vi "_CSMOFGV Dequeue.vi"(8 "Error In":errorcluster caption="error in (no error)", 9 "Dequeue Timeout (0ms)":i32, 10 "State (S) In (\"\")":string, 11 "CSMQ In":T1={"info"={"Module Name"="", "Requested Name"="", "Group Name"="", "Mode"=enum."Stand Alone", "Allowed Messages"=[]}, "Refs"={"WatchDogQ"=refnum, "CSMDataDVR"=refnum, "Queue"={"HPriorityQ"=refnum, "LowPriorityQ"=refnum}, "GroupDataDVR"=refnum, "TagMap"=refnum, "ExitEvent"=refnum, "NewStateEvent"=refnum, "StatusChangeEvent"=refnum}}) -> (0 "error out":errorcluster, 2 "States Out":string, 3 "CSMQ Out":T1={"info"={"Module Name"="", "Requested Name"="", "Group Name"="", "Mode"=enum."Stand Alone", "Allowed Messages"=[]}, "Refs"={"WatchDogQ"=refnum, "CSMDataDVR"=refnum, "Queue"={"HPriorityQ"=refnum, "LowPriorityQ"=refnum}, "GroupDataDVR"=refnum, "TagMap"=refnum, "ExitEvent"=refnum, "NewStateEvent"=refnum, "StatusChangeEvent"=refnum}})   [LabVIEW 2017, in "Communicable State Machine.lvlib"]
uses:
  Communicable State Machine.lvlib
  _CSMObj.ctl
  _CSMObj-Info.ctl
  Typedef/_CSM_MODE.ctl
  _CSMObj-Refs.ctl
  _CSMObj-Data.ctl
  Priority Queue/Priority Queue.ctl
  Typedef/_Cross CSM State Data.ctl
  Typedef/_CSM_MSG_TYPE.ctl
  Typedef/_Cross CSM State Response.ctl
  Typedef/_CSM_Response Source Message.ctl
  Priority Queue/def-Data(LowPRI-Q).ctl
  _CSMObj-ModeData.ctl
  Typedef/_CSM Status Change Event Data.ctl
  AdvanceAPI/CSM - Make String Arguments Safe.vi
  AdvanceAPI/CSM - Keywords.vi
  _Shared/CSM Shared.lvlib
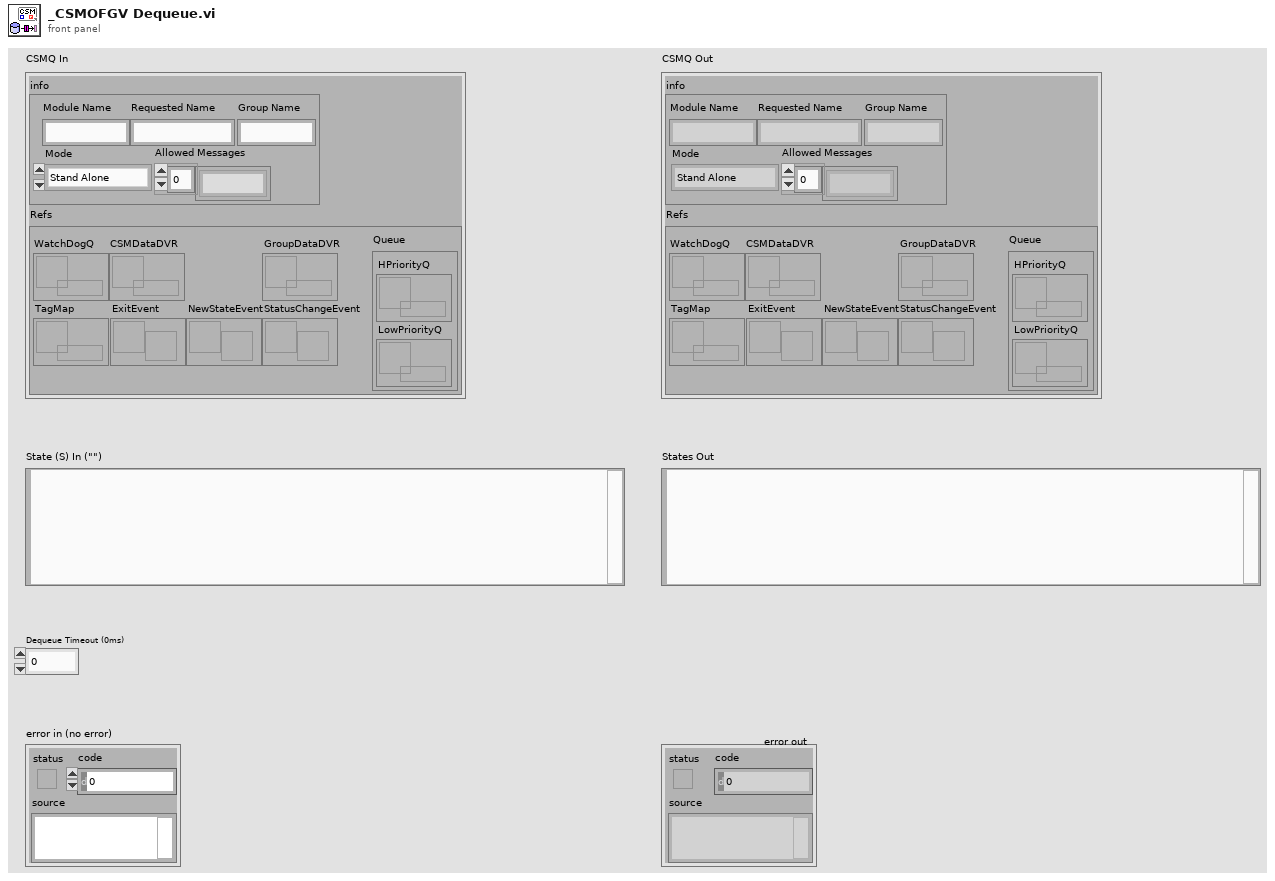
[diagram p1: front panel]
types:
  T1 = typedef "Communicable State Machine.lvlib/_CSMObj.ctl" = cluster{"info":T2, "Refs":T4}
  T2 = typedef "Communicable State Machine.lvlib/_CSMObj-Info.ctl" = cluster{"Module Name":string, "Requested Name":string, "Group Name":string, "Mode":T3, "Allowed Messages":string[]}
  T3 = typedef "Communicable State Machine.lvlib/_CSM_MODE.ctl" = enum16{"Not Exist", "Stand Alone", "CSM", "Worker", "Worker Agent", "Chain Node", "Chain"}
  T4 = typedef "Communicable State Machine.lvlib/_CSMObj-Refs.ctl" = cluster{"WatchDogQ":refnum<queue>, "CSMDataDVR":refnum<data-value>, "Queue":T5, "GroupDataDVR":refnum<data-value>, "TagMap":refnum<data-value>, "ExitEvent":refnum<user-event>, "NewStateEvent":refnum<user-event>, "StatusChangeEvent":refnum<user-event>}
  T5 = typedef "Communicable State Machine.lvlib/Priority Queue.ctl" = cluster{"HPriorityQ":refnum<queue>, "LowPriorityQ":refnum<queue>}
  T6 = typedef "Communicable State Machine.lvlib/_CSMObj-Data.ctl" = cluster{"RemoteMessge?":bool, "error":errorcluster, "InternalRegistryRules":string[], "Return State":string, "Initialized":enum16{"Initializing", "Ready", "Exiting"}}
  T7 = typedef "Communicable State Machine.lvlib/_Cross CSM State Data.ctl" = cluster{"Msg Type":T8, "state":string, "args":string, "source":string, "RespQ":refnum<queue>, "Response For Message":T9, "Target":string}
  T8 = typedef "Communicable State Machine.lvlib/_CSM_MSG_TYPE.ctl" = enum16{"Sync Message(-@)", "Async Message(->)", "Async without Response(->|)", "Async Response", "Broadcast(-><all>)", "Broadcast(-><status>)", "Broadcast(-><interrupt>)", "Append to JKISM States", "Append to JKISM States(High Priority)", "Broadcast(-><state>)"}
  T9 = typedef "Communicable State Machine.lvlib/_CSM_Response Source Message.ctl" = cluster{"‘State":string, "’Arguments":string, "’Error":errorcluster}
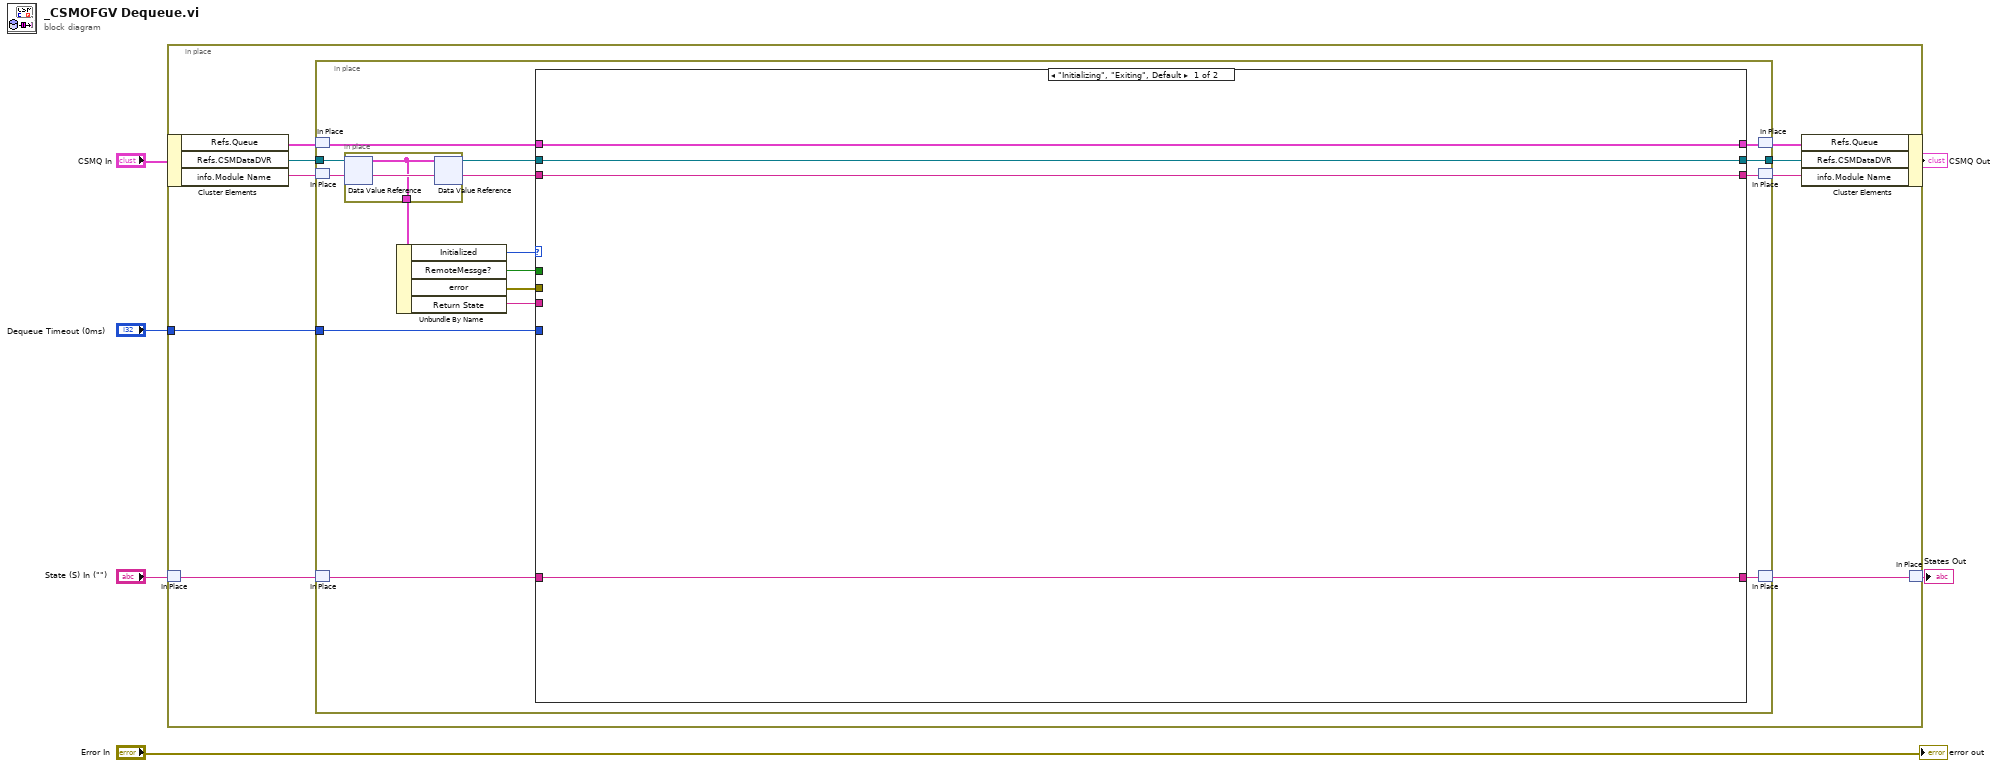
[diagram p0: block diagram]
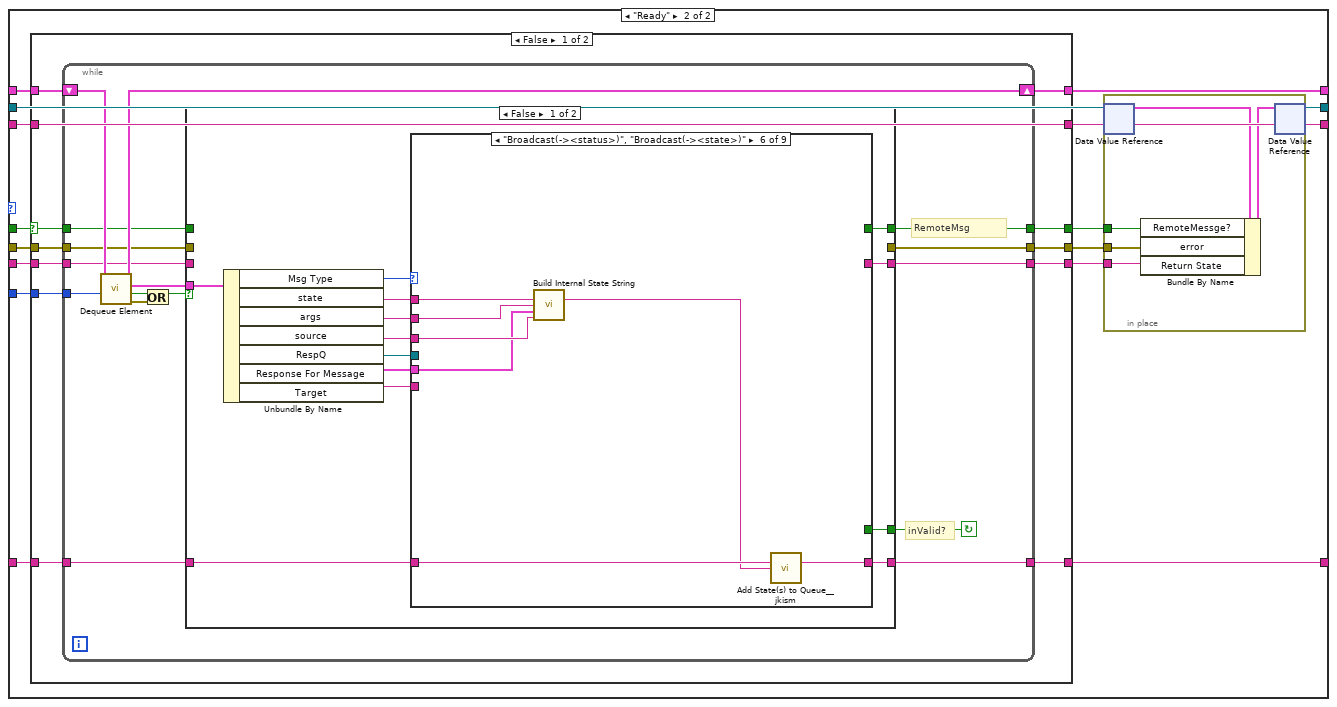
[diagram p2: hidden frame]
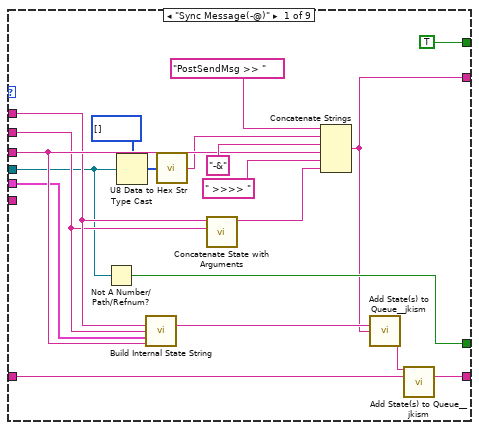
[diagram p3: hidden frame]
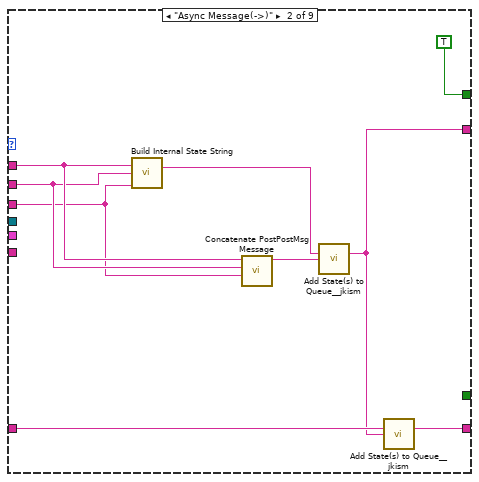
[diagram p4: hidden frame]
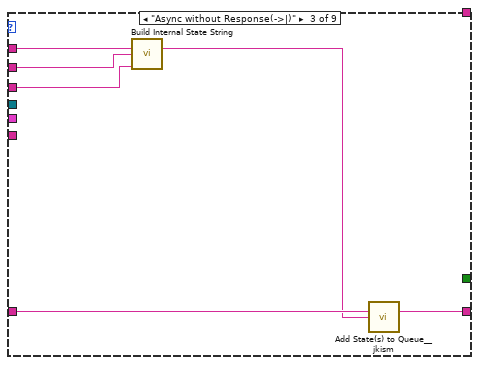
[diagram p5: hidden frame]
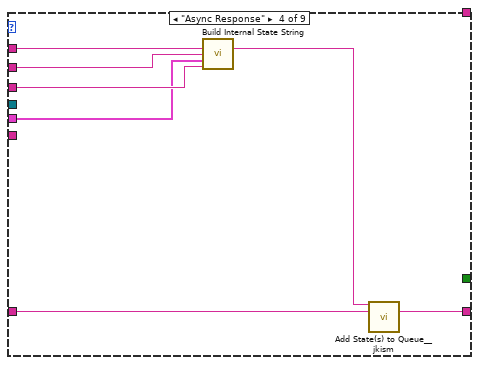
[diagram p6: hidden frame]
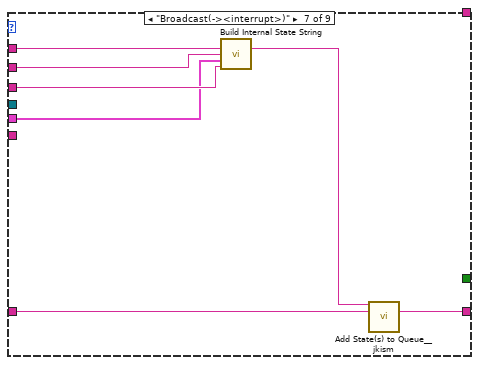
[diagram p8: hidden frame]
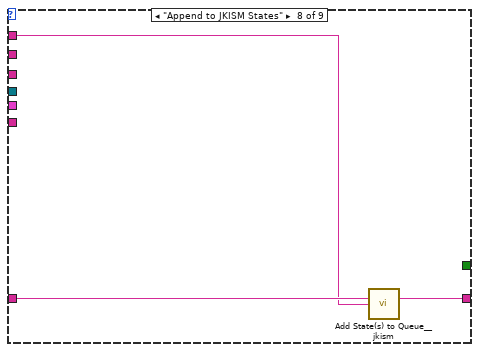
[diagram p9: hidden frame]
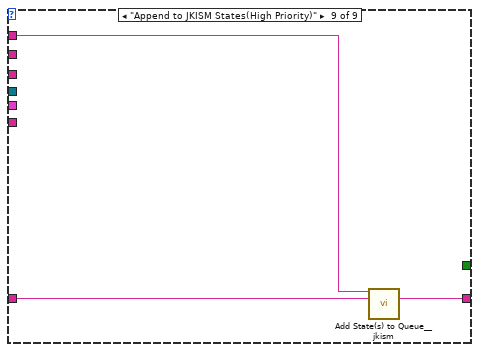
[diagram p10: hidden frame]
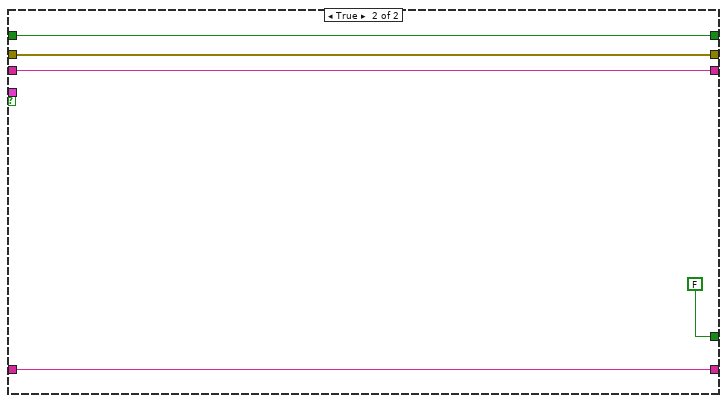
[diagram p11: hidden frame]
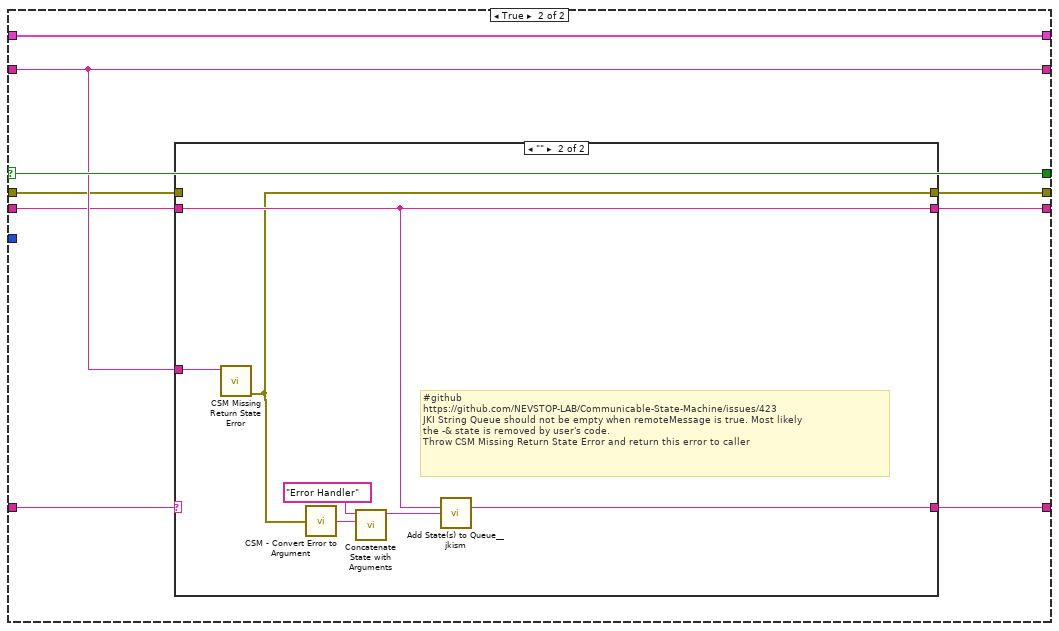
[diagram p12: hidden frame]
diagram:
  n1 = in-place "In Place Element Structure" {
    in-place-border: "Dequeue Timeout (0ms)" -> [w13]
    n2 = in-place-cluster #1("CSMQ In") -> ("Refs.Queue"=w15:T5, "Refs.CSMDataDVR"=w10:refnum<data-value>, "info.Module Name"=w7:string)
    n3 = in-place-match #2("State (S) In (\"\")") -> (w12:string)
    n4 = in-place {
      in-place-border: w13 -> [w28]
      in-place-border: w10 -> [w25]
      in-place-border: [w22] -> w9
      n5 = in-place-match #3(w15) -> (w29:T5)
      n6 = in-place-match #4(w7) -> (w18:string)
      n7 = in-place-match #5(w12) -> (w27:string)
      n8 = in-place {
        in-place-border: [w182] -> w24
        n9 = in-place-dvr #6(w25) -> (w182:T6)  [unwired: 1 out]
        n10 = in-place-dvr #6(w182) -> (w23:refnum<data-value>)  [unwired: 1 out]
      }
      n11 = Unbundle By Name(w24) -> ("Initialized"=w16:enum16{"Initializing", "Ready", "Exiting"}, "RemoteMessge?"=w21:bool, "error"=w20:errorcluster, "Return State"=w19:string)
      n12 = case shown="\"Initializing\", \"Exiting\", Default" w16 {
        tunnel: [w34 w49] -> w30
        tunnel: w29 -> [w34 w48]
        tunnel: w28 -> [_ w47]
        tunnel: w27 -> [w31 w46]
        tunnel: [w31 w45] -> w26
        tunnel: w23 -> [w33 w44]
        tunnel: [w33 w43] -> w22
        tunnel: w21 -> [_ w41]
        tunnel: w20 -> [_ w39]
        tunnel: w19 -> [_ w37]
        tunnel: w18 -> [w32 w36]
        tunnel: [w32 w35] -> w17
        frame "Initializing", "Exiting", Default {
        }
        frame "Ready" {
          n13 = case shown="False" w41 {
            selector: w41 -> [w60 w170]
            tunnel: [w65 w171] -> w49
            tunnel: w48 -> [w66 w171]
            tunnel: w47 -> [w64 _]
            tunnel: w46 -> [w63 w164]
            tunnel: [w62 w163] -> w45
            tunnel: [w61 w170] -> w42
            tunnel: [w59 w168] -> w40
            tunnel: w39 -> [w58 w167]
            tunnel: [w57 w166] -> w38
            tunnel: w37 -> [w56 w165]
            tunnel: w36 -> [w55 w169]
            tunnel: [w55 w169] -> w35
            frame False {
              n14 = while {
                tunnel: w64 -> [w80]
                shift-right: [w81] -> w65
                shift-left: w66 -> [w82]
                tunnel: w60 -> [w72]
                tunnel: [w73] -> w61
                tunnel: w63 -> [w78]
                tunnel: [w77] -> w62
                tunnel: [w70] -> w59
                tunnel: w58 -> [w69]
                tunnel: [w68] -> w57
                tunnel: w56 -> [w67]
                stop <- w71 continue-if-true
                # "inValid?"
                # "RemoteMsg"
                n15 = call "Dequeue Element.vi"("Timeout In ms (-1)"=w80, "Priority Queue"=w82) -> ("error out"=w74:errorcluster, "Timed Out?"=w75:bool, "Cross JKI State Machine State"=w79:T7, "Priority Queue (Dup)"=w81:T5)  [unwired: 5 in, 1 out]
                n16 = Or(x=w75, y=w74) -> (x .or. y?=w76:bool)
                n17 = case shown="False" w76 {
                  tunnel: w78 -> [w95 w162]
                  tunnel: [w94 w162] -> w77
                  tunnel: w79 -> [w89 _]
                  tunnel: [w85 w161] -> w73
                  tunnel: w72 -> [_ w161]
                  tunnel: [w84 FALSE] -> w71
                  tunnel: [_ w159] -> w70
                  tunnel: w69 -> [_ w159]
                  tunnel: [w83 w158] -> w68
                  tunnel: w67 -> [_ w158]
                  frame False {
                    n18 = Unbundle By Name(w89) -> ("Msg Type"=w87:T8, "state"=w92:string, "args"=w91:string, "source"=w90:string, "RespQ"=w93:refnum<queue>, "Response For Message"=w88:T9, "Target"=w86:string)
                    n19 = case shown="\"Broadcast(-><status>)\", \"Broadcast(-><state>)\"" w87 {
                      tunnel: w95 -> [w114 w123 w129 w136 w137 w144 w151 w154 w157]
                      tunnel: [w113 w122 w128 w135 w137 w143 w150 w153 w156] -> w94
                      tunnel: w93 -> [w98 _ _ _ _ _ _ _ _]
                      tunnel: w92 -> [w104 w118 w125 w132 _ w140 w147 w152 w155]
                      tunnel: w91 -> [w103 w117 w127 w134 _ w142 w149 _ _]
                      tunnel: w90 -> [w107 w116 w126 w133 _ w141 w148 _ _]
                      tunnel: w88 -> [w105 _ _ w130 _ w139 w146 _ _]
                      tunnel: w86 -> [_ _ _ _ _ _ _ _ _]
                      tunnel: [TRUE TRUE _ _ _ _ _ _ _] -> w85
                      tunnel: [w97 _ _ _ _ _ _ _ _] -> w84
                      tunnel: [w96 w119 _ _ _ _ _ _ _] -> w83
                      frame "Sync Message(-@)" {
                        n20 = Not A Number/Path/Refnum?(number/path/refnum=w98) -> (NaN/Path/Refnum?=w97:bool)
                        n21 = Type Cast(type=u8[] [], x=w98) -> (*(type *) &x=w100:u8[])
                        n22 = call "Build Internal State String.vi"("State"=w104, "Arguments (\"\")"=w103, ">> Response Source Message >>"=w105, "Source (\"\")"=w107) -> ("State With Arguments"=w110:string)  [unwired: 11 in]
                        n23 = call "U8 Data to Hex Str.vi"("U8 Data[]"=w100) -> ("HEX String (0-9,A-F)"=w99:string)
                        n24 = call "Concatenate State with Arguments.vi"("Arguments"=w103, "State"=w104) -> ("State With Arguements"=w102:string)  [unwired: 9 in]
                        n25 = Concatenate Strings("PostSendMsg >> " ("State(s) at Back (\"\")"), w99, "-&" ("string"), w107, " >>>> " ("string"), w102) -> (w96:string)
                        n26 = call "Add State(s) to Queue__jkism.vi"("State(s) in (\"\")"=w110, "State(s) at Back (\"\")"=w96) -> ("States Out"=w112:string)  [unwired: 13 in]
                        n27 = call "Add State(s) to Queue__jkism.vi"("State(s) in Front (\"\")"=w112, "State(s) in (\"\")"=w114) -> ("States Out"=w113:string)  [unwired: 13 in]
                      }
                      frame "Async Message(->)" {
                        n28 = call "Build Internal State String.vi"("State"=w118, "Arguments (\"\")"=w117, "Source (\"\")"=w116) -> ("State With Arguments"=w121:string)  [unwired: 12 in]
                        n29 = call "Concatenate PostPostMsg Message.vi"("Source"=w116, "Arguments"=w117, "Async-Message"=w118) -> ("PostPostMsg Message"=w115:string)  [unwired: 8 in]
                        n30 = call "Add State(s) to Queue__jkism.vi"("State(s) in (\"\")"=w121, "State(s) at Back (\"\")"=w115) -> ("States Out"=w119:string)  [unwired: 13 in]
                        n31 = call "Add State(s) to Queue__jkism.vi"("State(s) in (\"\")"=w123, "State(s) at Back (\"\")"=w119) -> ("States Out"=w122:string)  [unwired: 13 in]
                      }
                      frame "Async without Response(->|)" {
                        n32 = call "Build Internal State String.vi"("State"=w125, "Arguments (\"\")"=w127, "Source (\"\")"=w126) -> ("State With Arguments"=w124:string)  [unwired: 12 in]
                        n33 = call "Add State(s) to Queue__jkism.vi"("State(s) in (\"\")"=w129, "State(s) at Back (\"\")"=w124) -> ("States Out"=w128:string)  [unwired: 13 in]
                      }
                      frame "Async Response" {
                        n34 = call "Build Internal State String.vi"("State"=w132, "Arguments (\"\")"=w134, ">> Response Source Message >>"=w130, "Source (\"\")"=w133) -> ("State With Arguments"=w131:string)  [unwired: 11 in]
                        n35 = call "Add State(s) to Queue__jkism.vi"("State(s) in Front (\"\")"=w131, "State(s) in (\"\")"=w136) -> ("States Out"=w135:string)  [unwired: 13 in]
                      }
                      frame "Broadcast(-><all>)" {
                        # "#CSM-NOTE\nshould no be here"
                      }
                      frame "Broadcast(-><status>)", "Broadcast(-><state>)" {
                        n36 = call "Build Internal State String.vi"("State"=w140, "Arguments (\"\")"=w142, ">> Response Source Message >>"=w139, "Source (\"\")"=w141) -> ("State With Arguments"=w138:string)  [unwired: 11 in]
                        n37 = call "Add State(s) to Queue__jkism.vi"("State(s) in (\"\")"=w144, "State(s) at Back (\"\")"=w138) -> ("States Out"=w143:string)  [unwired: 13 in]
                      }
                      frame "Broadcast(-><interrupt>)" {
                        n38 = call "Build Internal State String.vi"("State"=w147, "Arguments (\"\")"=w149, ">> Response Source Message >>"=w146, "Source (\"\")"=w148) -> ("State With Arguments"=w145:string)  [unwired: 11 in]
                        n39 = call "Add State(s) to Queue__jkism.vi"("State(s) in Front (\"\")"=w145, "State(s) in (\"\")"=w151) -> ("States Out"=w150:string)  [unwired: 13 in]
                      }
                      frame "Append to JKISM States" {
                        n40 = call "Add State(s) to Queue__jkism.vi"("State(s) in (\"\")"=w154, "State(s) at Back (\"\")"=w152) -> ("States Out"=w153:string)  [unwired: 13 in]
                      }
                      frame "Append to JKISM States(High Priority)" {
                        n41 = call "Add State(s) to Queue__jkism.vi"("State(s) in Front (\"\")"=w155, "State(s) in (\"\")"=w157) -> ("States Out"=w156:string)  [unwired: 13 in]
                      }
                    }
                  }
                  frame True {
                  }
                }
              }
            }
            frame True {
              n42 = case shown="\"\"" w164 {
                selector: w164 -> [w172 _]
                tunnel: w169 -> [_ w181]
                tunnel: [w174 w176] -> w168
                tunnel: w167 -> [w174 _]
                tunnel: [w173 w179] -> w166
                tunnel: w165 -> [w173 w179]
                tunnel: [w172 w180] -> w163
                frame Default {
                }
                frame "" {
                  # "#github \nhttps://github.com/NEVSTOP-LAB/Communicable-State-Machine/issues/423\nJKI String Queue should not be empty when remoteMessage is true. Most likely\nthe -& state is removed by user's code. \nThrow CSM Missing Return State Error and return this error to caller"
                  n43 = call "CSM Missing Return State Error.vi"("Arguments (As CSM Name)"=w181) -> ("error out"=w176:errorcluster)  [unwired: 10 in]
                  n44 = call "CSM - Convert Error to Argument.vi"("Error"=w176) -> ("Argument"=w177:string)  [unwired: 4 in]
                  n45 = call "Concatenate State with Arguments.vi"("Arguments"=w177, "State"="Error Handler") -> ("State With Arguements"=w178:string)  [unwired: 9 in]
                  n46 = call "Add State(s) to Queue__jkism.vi"("State(s) in (\"\")"=w179, "State(s) at Back (\"\")"=w178) -> ("States Out"=w180:string)  [unwired: 13 in]
                }
              }
            }
          }
          n47 = in-place {
            in-place-border: w42 -> [w52]
            in-place-border: w40 -> [w51]
            in-place-border: w38 -> [w50]
            n48 = in-place-dvr #7(w44) -> (w54:T6)  [unwired: 1 out]
            n49 = Bundle By Name(cluster=w54, "RemoteMessge?"=w52, "error"=w51, "Return State"=w50) -> (w53:T6)
            n50 = in-place-dvr #7(w53) -> (w43:refnum<data-value>)  [unwired: 1 out]
          }
        }
      }
      n51 = in-place-match #3(w30) -> (w14:T5)
      n52 = in-place-match #4(w17) -> (w8:string)
      n53 = in-place-match #5(w26) -> (w11:string)
    }
    n54 = in-place-cluster #1("Refs.Queue"=w14, "Refs.CSMDataDVR"=w9, "info.Module Name"=w8) -> (→"CSMQ Out":T1)
    n55 = in-place-match #2(w11) -> (→"States Out":string)
  }
  "error out" <- "Error In"
